vi "Set Item Test.vi"() -> ()   [LabVIEW 2017]
uses:
  JSONtext.lvlib
  <vilib>/addons/_JKI Toolkits/Caraya/classes/Assert/Assert.lvclass
  <vilib>/addons/_JKI Toolkits/Caraya/classes/Test/Test.lvclass
panel:
  out "error out":errorcluster
  out "Array 2":string[](array[string])
  out "Array":bool[](array[boolean])
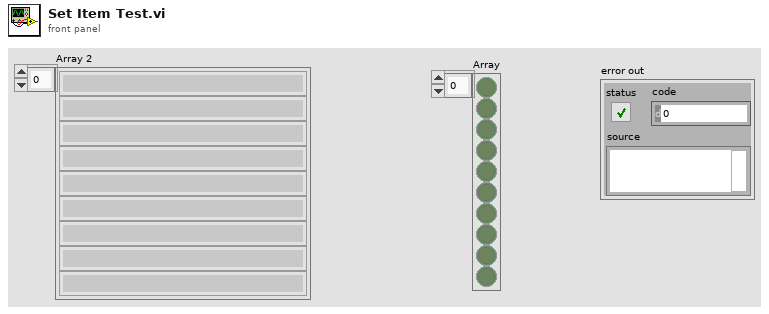
[diagram p1: front panel]
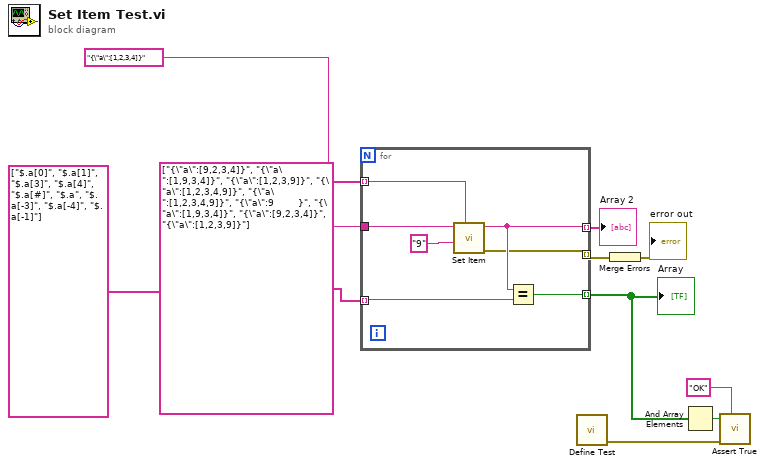
[diagram p0: block diagram]
diagram:
  n1 = for {
    tunnel: "{\"a\":[1,2,3,4]}" -> [w17]
    tunnel: string[] ["$.a[0]", "$.a[1]", "$.a[3]", "$.a[4]", "$.a[#]", "$.a", "$.a[-3]", "$.a[-4]", "$.a[-1]"] -> [w16] mode=indexing
    tunnel: string[] ["{\"a\":[9,2,3,4]}", "{\"a\":[1,9,3,4]}", "{\"a\":[1,2,3,9]}", "{\"a\":[1,2,3,4,9]}", "{\"a\":[1,2,3,4,9]}", "{\"a\":9        }", "{\"a\":[1,9,3,4]}", "{\"a\":[9,2,3,4]}", "{\"a\":[1,2,3,9]}"] -> [w15] mode=indexing
    tunnel: [w14] -> w3 mode=indexing
    tunnel: [w12] -> w7 mode=indexing
    tunnel: [w11] -> w2 mode=indexing
    n2 = call "Set Item.vi"("$Path or Item Name"=w16, "JSON to Insert"="9", "JSON"=w17) -> ("error out"=w11:errorcluster, "<JSON>"=w12:string)  [unwired: 5 in, 1 out]
    n3 = Equal?(x=w12, y=w15) -> (x = y?=w14:bool)
  }
  "Array" <- w3
  "Array 2" <- w7
  n4 = call <vilib>:"Define Test.vi"() -> ("error out"=w4:errorcluster)  [unwired: 11 in]
  n5 = Merge Errors(w2) -> (→"error out":errorcluster)
  n6 = And Array Elements(Boolean array=w3) -> (logical AND=w6:bool)
  n7 = call <vilib>:"Assert True.vi"("Label"="OK", "error in (no error)"=w4, "True?"=w6) -> ()  [unwired: 8 in, 1 out]
